vi "PSVCH_Get Data.vi"(8 "Error In (no error)":errorcluster, 10 "Time Out(10)":i32=10, 11 "ChlName":string) -> (0 "Error Out":errorcluster, 2 "timed out?":bool, 3 "Data":waveform(dbl))   [LabVIEW 2016]
panel:
  # "Data Out"
  # "Data In"
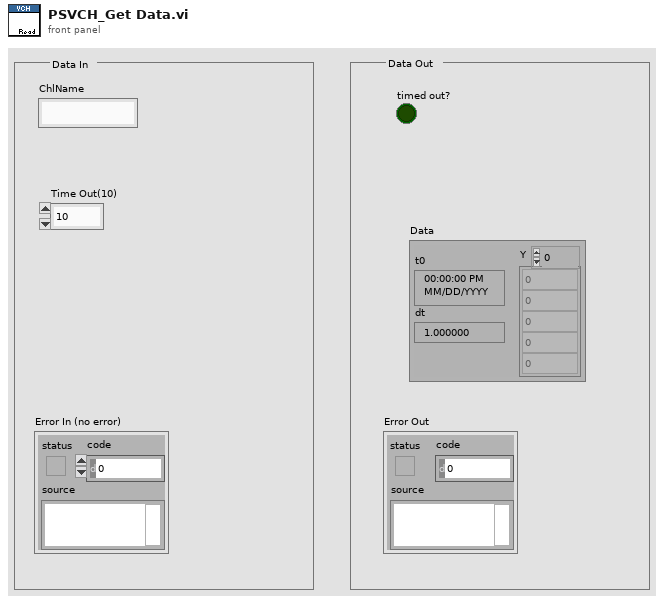
[diagram p1: front panel]
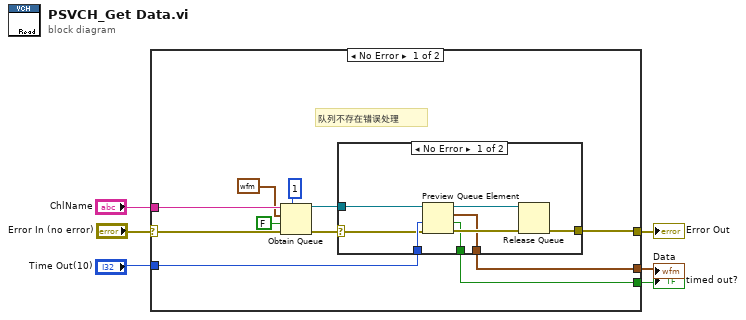
[diagram p0: block diagram]
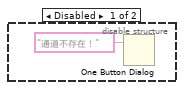
[diagram p3: hidden frame]
diagram:
  n1 = case shown="No Error" "Error In (no error)" {
    selector: "Error In (no error)" -> [w14 w27]
    tunnel: [w15 w27] -> w5
    tunnel: "ChlName" -> [w13 _]
    tunnel: "Time Out(10)" -> [w12 _]
    tunnel: [w11 _] -> w2
    tunnel: [w10 _] -> w1
    frame No Error {
      # "队列不存在错误处理"
      n2 = Obtain Queue(max queue size (-1, unlimited)=1 ("队列最大值（-1，无限）"), name (unnamed)=w13, element data type=waveform(dbl) {"t0"=timestamp(0 s since 1904-01-01), "dt"=1.0, "Y"=[]} ("Waveform"), create if not found? (T)=FALSE ("如未找到是否创建？(T)"), error in (no error)=w14) -> (queue out=w17:refnum<queue>, error out=w9:errorcluster)  [unwired: 1 out]
      n3 = case shown="No Error" w9 {
        selector: w9 -> [w18 _]
        tunnel: w17 -> [w23 _]
        tunnel: [w22 _] -> w15
        tunnel: w12 -> [w21 _]
        tunnel: [w20 _] -> w11
        tunnel: [w19 _] -> w10
        frame No Error {
          n4 = Preview Queue Element(queue=w23, timeout in ms (-1)=w21, error in (no error)=w18) -> (queue out=w24:refnum<queue>, element=w20:waveform(dbl), timed out?=w19:bool, error out=w25:errorcluster)
          n5 = Release Queue(queue=w24, error in (no error)=w25) -> (error out=w22:errorcluster)  [unwired: 1 in, 2 out]
        }
        frame Error {
          n6 = disable-structure shown="启用" {
            frame Disabled {
              n7 = One Button Dialog(message="通道不存在！") -> ()  [unwired: 1 in, 1 out]
            }
            frame Enabled {
            }
          }
        }
      }
    }
    frame Error {
    }
  }
  "Error Out" <- w5
  "Data" <- w2
  "timed out?" <- w1
